vi "Setup Columns.vi"(8 "error in (no error)":errorcluster, 10 "ColumnSetup":T1[](array[typedef]) {"MinWidth" min=2 step=1; "AutoSizeMode" items=["None"=1, "ColumnHeader"=2, "AllCellsExceptHeader"=4, "AllCells"=6, "DisplayedCellsExceptHeader"=8, "DisplayedCells"=10, "Fill"=16]; "FillWeight" min=1 max=100}, 11 "DataGridViewColumnCollection":refnum<k24>) -> (0 "error out":errorcluster)   [LabVIEW 2014, in "DataGridView.lvclass"]
uses:
  DataGridView.lvclass
  System.Windows.Forms
  GridColumn/ColumnDefinition.ctl
  GridColumn/GridColumn.lvclass
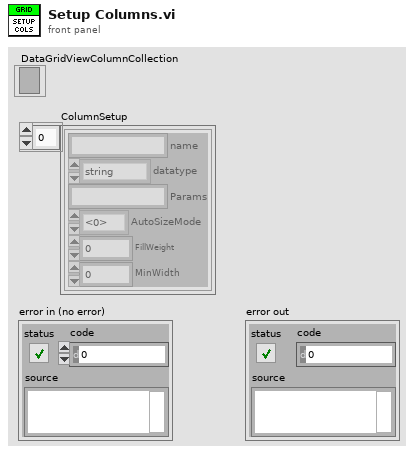
[diagram p1: front panel]
types:
  T1 = typedef "GridColumn.lvclass/ColumnDefinition.ctl" = cluster{"name":string, "datatype":enum16{"string", "image", "check", "numeric", "timestamp", "button", "combo"}, "Params":string, "AutoSizeMode":i32, "FillWeight":sgl, "MinWidth":i32}
  T2 = enum16{"string", "image", "check", "numeric", "timestamp", "button", "combo"}
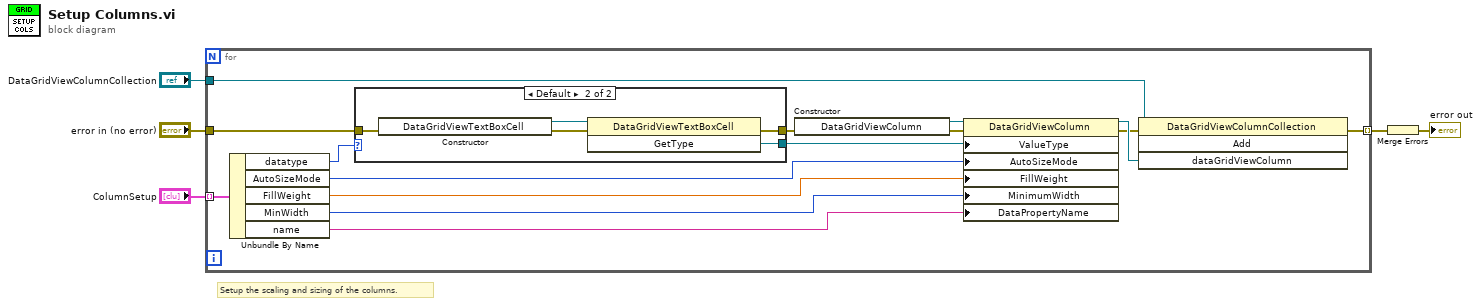
[diagram p0: block diagram]
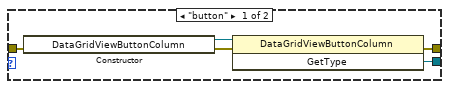
[diagram p2: hidden frame]
diagram:
  # "Setup the scaling and sizing of the columns."
  n1 = for {
    tunnel: "ColumnSetup" -> [w19] mode=indexing
    tunnel: "error in (no error)" -> [w18]
    tunnel: [w8] -> w4 mode=indexing
    tunnel: "DataGridViewColumnCollection" -> [w15]
    n2 = Unbundle By Name(w19) -> ("datatype"=w13:T2, "AutoSizeMode"=w12:i32, "FillWeight"=w11:sgl, "MinWidth"=w10:i32, "name"=w6:string)
    n3 = case shown="Default" w13 {
      tunnel: [w20 w25] -> w7
      tunnel: w18 -> [w22 w27]
      tunnel: [w21 w26] -> w14
      frame "button" {
        n4 = constructor class="DataGridViewButtonColumn"(error in=w22) -> (reference out=w24:refnum<k24>, error out=w23:errorcluster)  [unwired: 2 in, 1 out]
        n5 = invoke class="DataGridViewButtonColumn" method="GetType"(reference=w24, error in=w23) -> (error out=w20:errorcluster, "GetType"=w21:refnum<k24>)  [unwired: 1 in, 1 out]
      }
      frame Default {
        n6 = constructor class="DataGridViewTextBoxCell"(error in=w27) -> (reference out=w29:refnum<k24>, error out=w28:errorcluster)  [unwired: 2 in, 1 out]
        n7 = invoke class="DataGridViewTextBoxCell" method="GetType"(reference=w29, error in=w28) -> (error out=w25:errorcluster, "GetType"=w26:refnum<k24>)  [unwired: 1 in, 1 out]
      }
    }
    n8 = constructor class="DataGridViewColumn"(error in=w7) -> (reference out=w9:refnum<k24>, error out=w8:errorcluster)  [unwired: 2 in, 1 out]
    n9 = property class="DataGridViewColumn"(reference=w9, "ValueType"=w14, "AutoSizeMode"=w12, "FillWeight"=w11, "MinimumWidth"=w10, "DataPropertyName"=w6) -> (reference out=w17:refnum<k24>, error out=w16:errorcluster)  [unwired: 1 in]
    n10 = invoke class="DataGridViewColumnCollection" method="Add"(reference=w15, error in=w16, "dataGridViewColumn"=w17) -> ()  [unwired: 1 in, 4 out]
  }
  n11 = Merge Errors(w4) -> (→"error out":errorcluster)
